vi "FTW-File-ResourceDirectory.vi"(11 "error in":errorcluster) -> (4 "LabVIEW":path, 6 "Resource":path, 8 "Providers":path, 10 "Provider API":path, 15 "error out":errorcluster)   [LabVIEW 2015]
panel:
  # "Inputs"
  # "Outputs"
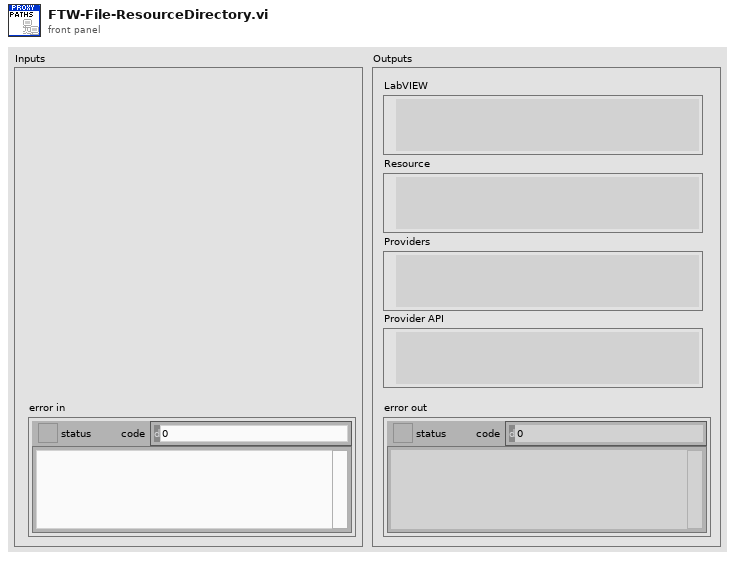
[diagram p1: front panel]
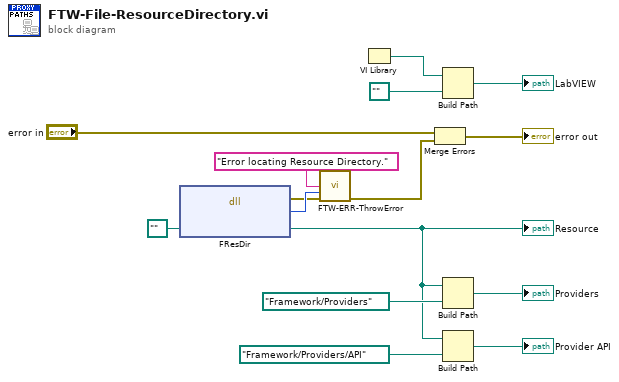
[diagram p0: block diagram]
diagram:
  n1 = dll-call lib="LabVIEW" fn="FResDir"("Resource Directory"=path "") -> (error out=w5:errorcluster, "Error"=w6:i32, "Resource Directory"=w7:path)  [unwired: 3 in, 1 out]
  "Resource" <- w7
  n2 = call "FTW-ERR-ThrowError.vi"("Error Message"="Error locating Resource Directory.", "Error Code"=w6, "error in"=w5) -> ("error out"=w2:errorcluster)  [unwired: 12 in]
  n3 = VI Library() -> (path=w12:path)
  n4 = Merge Errors("error in", w2) -> (→"error out":errorcluster)
  n5 = Build Path(base path=w12, name or relative path=path "..") -> (appended path=→"LabVIEW":path)
  n6 = Build Path(base path=w7, name or relative path=path "Framework/Providers") -> (appended path=→"Providers":path)
  n7 = Build Path(base path=w7, name or relative path=path "Framework/Providers/API") -> (appended path=→"Provider API":path)
